vi "Pythagoras.vi"() -> ()   [LabVIEW 2017]
panel:
  out "c":dbl
  in  "b2":dbl
  in  "a":dbl
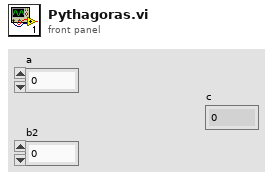
[diagram p1: front panel]
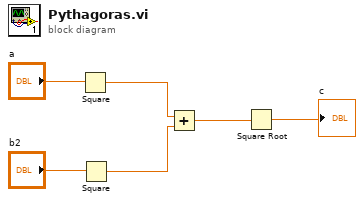
[diagram p0: block diagram]
diagram:
  n1 = Square(x="a") -> (x^2=w3:dbl)
  n2 = Square(x="b2") -> (x^2=w4:dbl)
  n3 = Add(x=w3, y=w4) -> (x+y=w2:dbl)
  n4 = Square Root(x=w2) -> (sqrt(x)=→"c":dbl)
